vi "GetOutputWireBranch.vi"(6 "error in":errorcluster, 9 "Tunnel in":refnum<class "Tunnel.lvclass">) -> (0 "error out":errorcluster, 3 "Tunnel out":refnum<class "Tunnel.lvclass">, 4 "branches":string, 5 "branched":bool)   [LabVIEW 2014, in "Raspberry Pi Compatible Compiler for LabVIEW.lvlib" / "Tunnel.lvclass"]
uses:
  Tunnel.lvclass
  Tunnel.lvclass/Tunnel.ctl
  Terminal/Terminal.lvclass
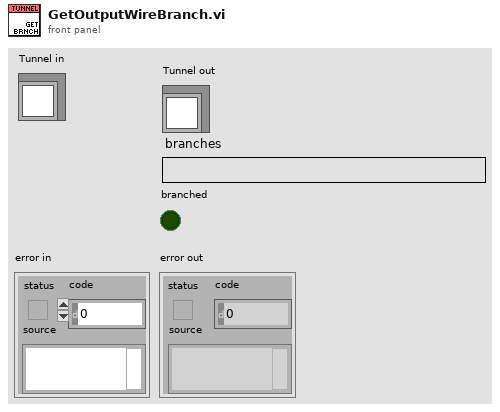
[diagram p1: front panel]
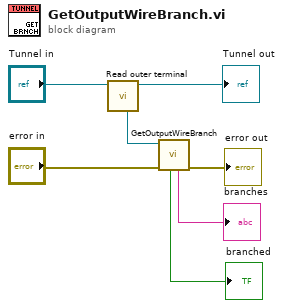
[diagram p0: block diagram]
diagram:
  n1 = call "Read outer terminal.vi"("Tunnel in"="Tunnel in") -> ("Tunnel out"=→"Tunnel out":refnum<class "Tunnel.lvclass">, "outer terminal"=w6:refnum<class "Terminal.lvclass">)  [unwired: 7 in]
  n2 = call-dynamic "GetOutputWireBranch.vi"("error in"="error in", "Terminal in"=w6) -> ("error out"=→"error out":errorcluster, "branches"=→"branches":string, "branched"=→"branched":bool)  [unwired: 4 in, 1 out]
